vi "WakeUpHeatCamera(SubVI).vi"(10 "Time (ms) to wait":dbl=20000.0) -> ()   [LabVIEW 2020]
uses:
  <vilib>/httpClient/LabVIEWHTTPClient.lvlib
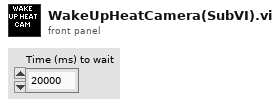
[diagram p1: front panel]
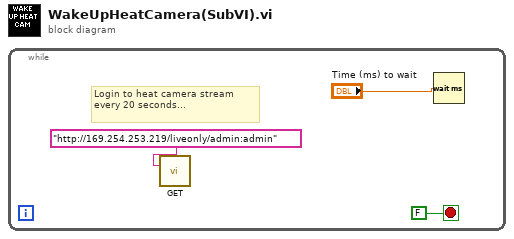
[diagram p0: block diagram]
diagram:
  n1 = while {
    stop <- FALSE stop-if-true
    # "Login to heat camera stream every 20 seconds..."
    n2 = call <vilib>:"GET.vi"("url"="http://169.254.253.219/liveonly/admin:admin") -> ()  [unwired: 11 in, 4 out]
    n3 = Wait (ms)(milliseconds to wait="Time (ms) to wait") -> ()  [unwired: 1 out]
  }
